vi "IO_csv_writer.vi"(0 "info_sheet":string, 1 "path":string, 2 "y_data_arr":dbl[][](array[numeric]), 3 "x_data_arr":dbl[][](array[numeric])) -> ()   [LabVIEW 2014]
uses:
  dll/csv_operator.dll
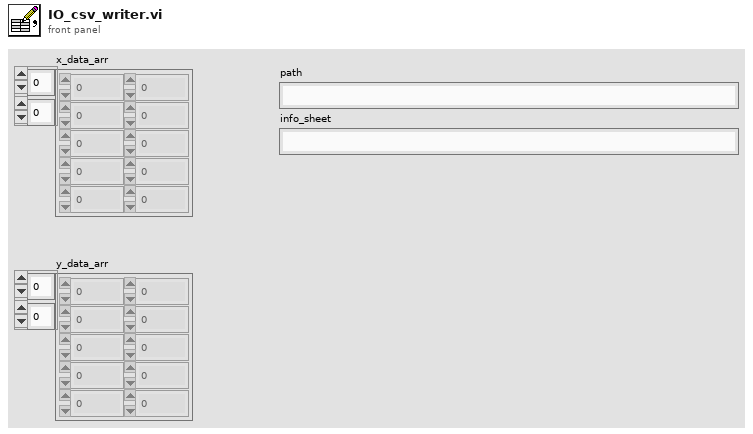
[diagram p1: front panel]
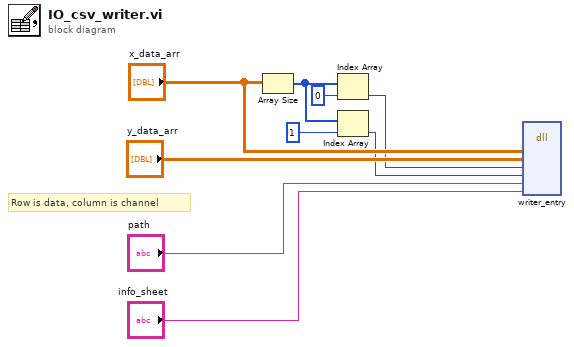
[diagram p0: block diagram]
diagram:
  # "Row is data, column is channel"
  n1 = Array Size(array="x_data_arr") -> (size(s)=w3:i32[])
  n2 = Index Array(array=w3, index=0) -> (element=w2:i32)
  n3 = Index Array(array=w3, index=1) -> (element=w1:i32)
  n4 = dll-call lib="C:/Users/DrippySummer/Documents/LabVIEW Data/SavaData/keithley_general_client/dll/csv_operator.dll" fn="writer_entry"("x_data_array"="x_data_arr", "y_data_array"="y_data_arr", "row_num"=w2, "col_num"=w1, "path"="path", "info_sheet"="info_sheet") -> ()  [unwired: 10 in, 2 out]
